vi "Default Instrument Setup.vi"(8 "error in (no error)":errorcluster, 11 "VISA resource name":refnum<visa-resource-name>) -> (0 "error out":errorcluster, 3 "VISA resource name out":refnum<visa-resource-name>)   [LabVIEW 2015, in "Tektronix DPO MSO 2000 4000 Series.lvlib"]
doc: "This Utility VI sends a default command string to the instrument whenever a new VISA session is opened, or the instrument is reset. Use this VI as a subVI for the <B>Initialize</B> and <B>Reset</B> VIs. Altering this VI could cause these two VIs to operate incorrectly."
uses:
  Tektronix DPO MSO 2000 4000 Series.lvlib
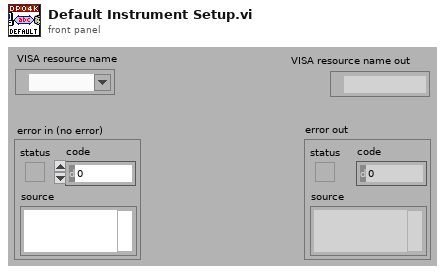
[diagram p1: front panel]
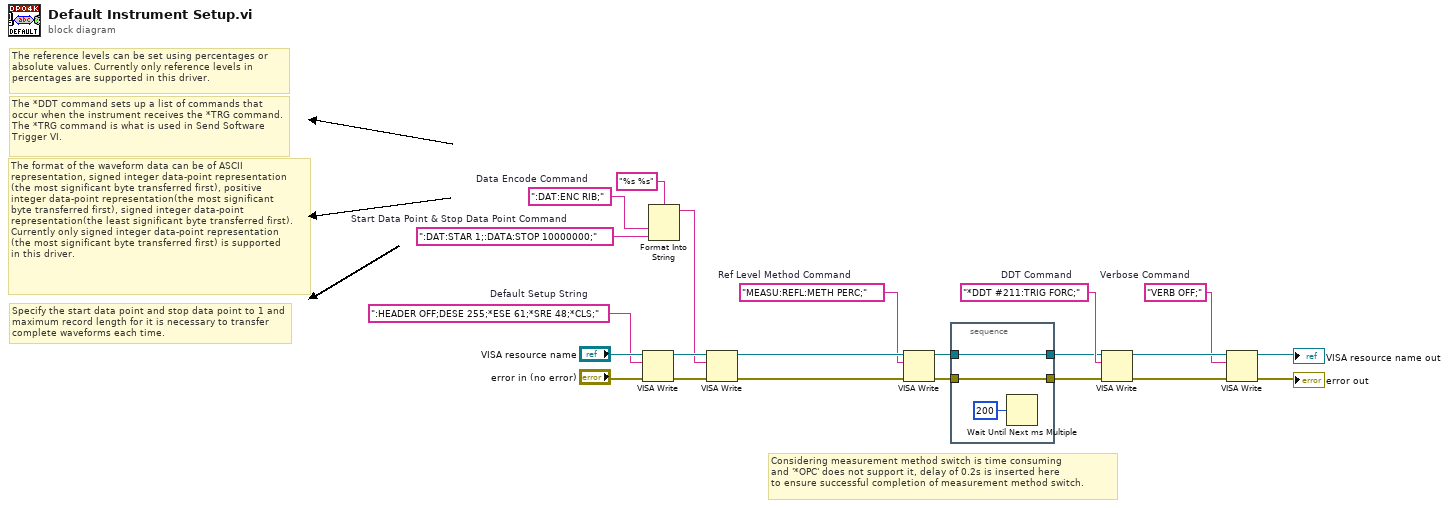
[diagram p0: block diagram]
diagram:
  w3 = "MEASU:REFL:METH PERC;"  # Ref Level Method Command
  w10 = "VERB OFF;"  # Verbose Command
  w15 = "*DDT #211:TRIG FORC;"  # DDT Command
  w9 = ":DAT:ENC RIB;"  # Data Encode Command
  w8 = ":DAT:STAR 1;:DATA:STOP 10000000;"  # Start Data Point & Stop Data Point Command
  w20 = ":HEADER OFF;DESE 255;*ESE 61;*SRE 48;*CLS;"  # Default Setup String
  # "Considering measurement method switch is time consuming\nand '*OPC' does not support it, delay of 0.2s is inserted here \nto ensure successful completion of measurement method switch."
  # "Specify the start data point and stop data point to 1 and maximum record length for it is necessary to transfer complete waveforms each time."
  # "The format of the waveform data can be of ASCII\nrepresentation, signed integer data-point representation\n(the most significant byte transferred first), positive \ninteger data-point representation(the most significant \nbyte transferred first), signed integer data-point \nrepresentation(the least significant byte transferred first).\nCurrently only signed integer data-point representation\n(the most significant byte transferred first) is supported\nin this driver."
  # "The reference levels can be set using percentages or absolute values. Currently only reference levels in \npercentages are supported in this driver."
  # "The *DDT command sets up a list of commands that occur when the instrument receives the *TRG command.  \nThe *TRG command is what is used in Send Software Trigger VI."
  n1 = VISA Write(VISA resource name="VISA resource name", write buffer=w20, error in (no error)="error in (no error)") -> (VISA resource name out=w19:refnum<visa-resource-name>, error out=w18:errorcluster)  [unwired: 1 out]
  n2 = Format Into String(format string="%s %s", w9, w8) -> (resulting string=w17:string)  [unwired: 2 in, 1 out]
  n3 = VISA Write(VISA resource name=w19, write buffer=w17, error in (no error)=w18) -> (VISA resource name out=w4:refnum<visa-resource-name>, error out=w5:errorcluster)  [unwired: 1 out]
  n4 = VISA Write(VISA resource name=w4, write buffer=w3, error in (no error)=w5) -> (VISA resource name out=w7:refnum<visa-resource-name>, error out=w6:errorcluster)  [unwired: 1 out]
  n5 = stacked-sequence {
    tunnel: w7 -> [w24]
    tunnel: [w24] -> w2
    tunnel: w6 -> [w23]
    tunnel: [w23] -> w1
    frame #0 {
      n6 = Wait Until Next ms Multiple(millisecond multiple=u32 200) -> ()  [unwired: 1 out]
    }
  }
  n7 = VISA Write(VISA resource name=w2, write buffer=w15, error in (no error)=w1) -> (VISA resource name out=w14:refnum<visa-resource-name>, error out=w13:errorcluster)  [unwired: 1 out]
  n8 = VISA Write(VISA resource name=w14, write buffer=w10, error in (no error)=w13) -> (VISA resource name out=→"VISA resource name out":refnum<visa-resource-name>, error out=→"error out":errorcluster)  [unwired: 1 out]
